vi "Basic Call Method.vi"(8 "Error In":errorcluster, 10 "args":string, 11 "method":string) -> (0 "Error Out":errorcluster, 3 "concatened string":string)   [LabVIEW 2014]
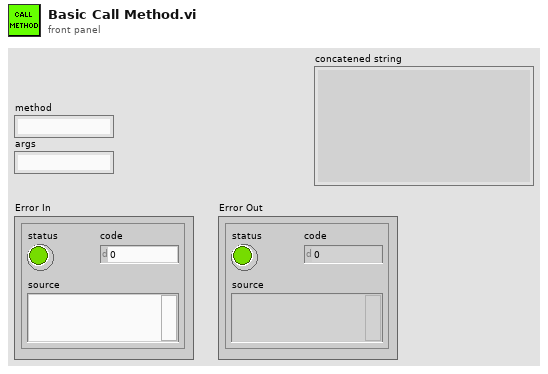
[diagram p1: front panel]
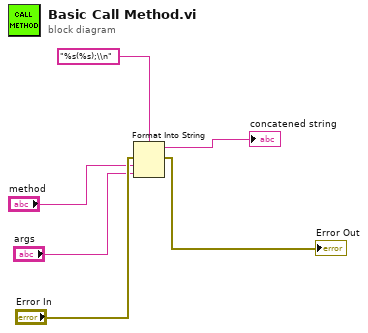
[diagram p0: block diagram]
diagram:
  n1 = Format Into String(format string="%s(%s);\\n", error in="Error In", "method", "args") -> (resulting string=→"concatened string":string, error out=→"Error Out":errorcluster)  [unwired: 1 in]
